vi "Event Handle Loop_Search Index.vi"(8 "error in (no error)":errorcluster, 10 "Coords":T1, 11 "QMenu Class in":refnum<class "QMenu Class.lvclass">) -> (0 "error out":errorcluster, 2 "Index":i32, 3 "QMenu Class out":refnum<class "QMenu Class.lvclass">)   [LabVIEW 2020, in "QTab.lvlib" / "QMenu Class.lvclass"]
uses:
  QMenu Class.lvclass
  <vilib>/Utility/miscctls.llb/LVPoint32TypeDef.ctl
  QMenu Class.lvclass/QMenu Class.ctl
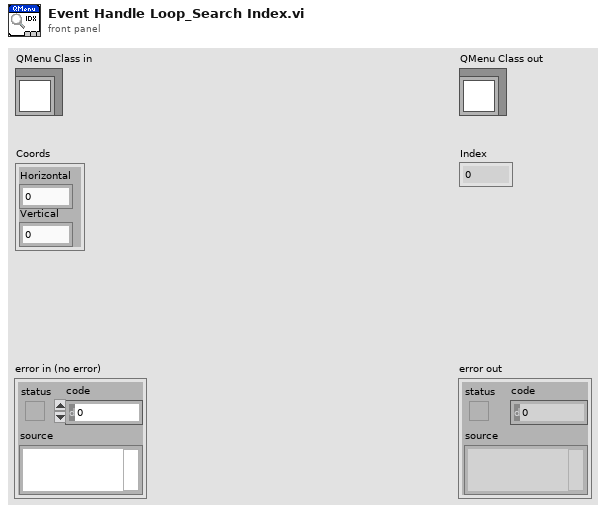
[diagram p1: front panel]
types:
  T1 = typedef "LVPoint32TypeDef.ctl" = cluster{"Horizontal":i32, "Vertical":i32}
  T2 = typedef "LVPositionTypeDef.ctl" = cluster{"Left":i32, "Top":i32}
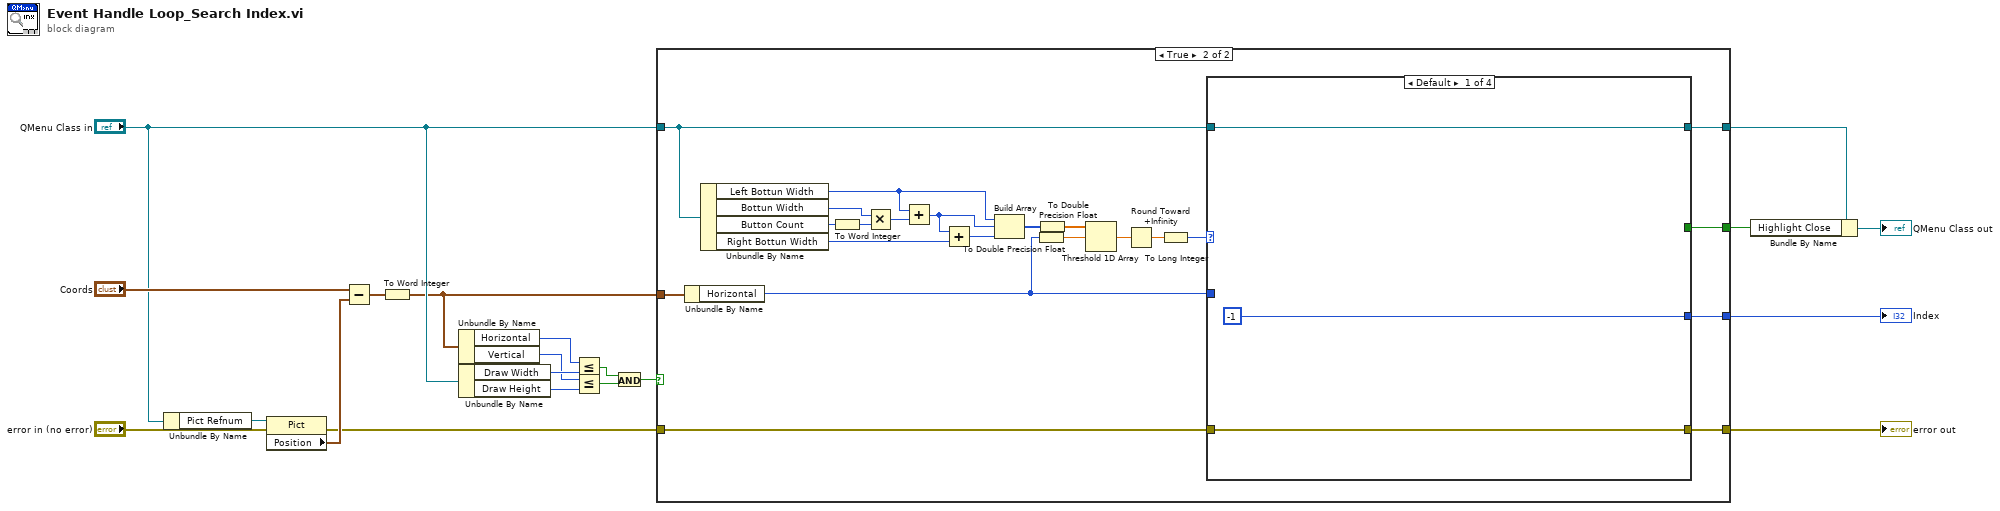
[diagram p0: block diagram]
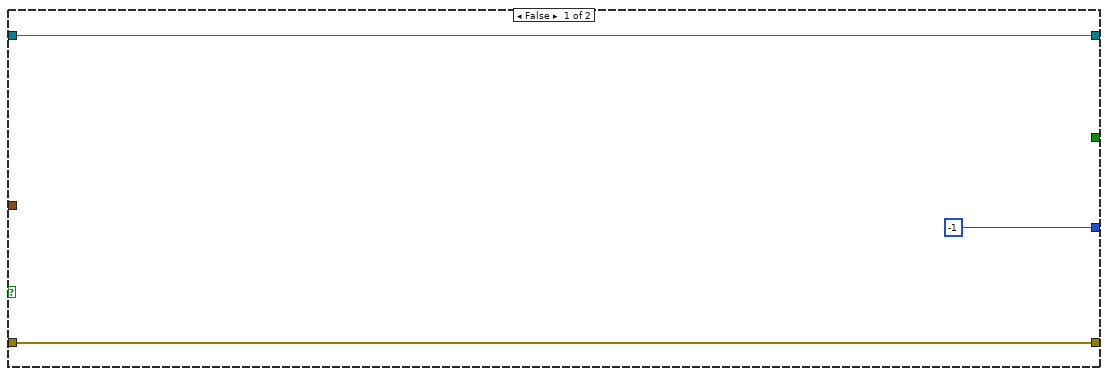
[diagram p2: hidden frame]
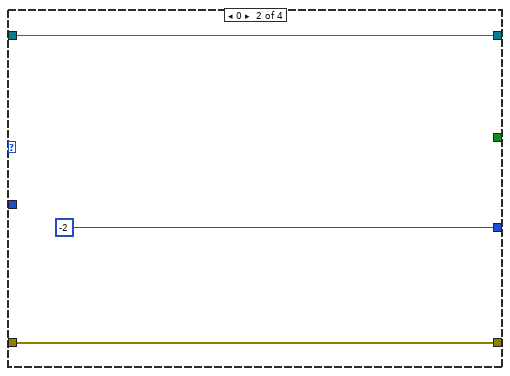
[diagram p3: hidden frame]
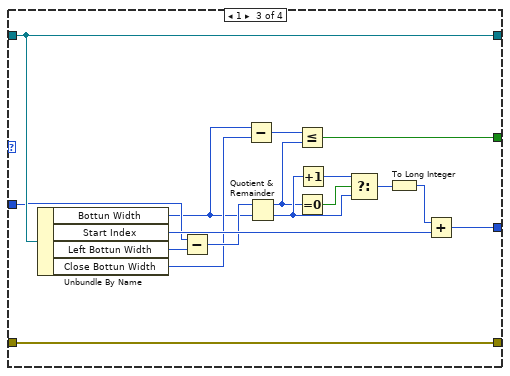
[diagram p4: hidden frame]
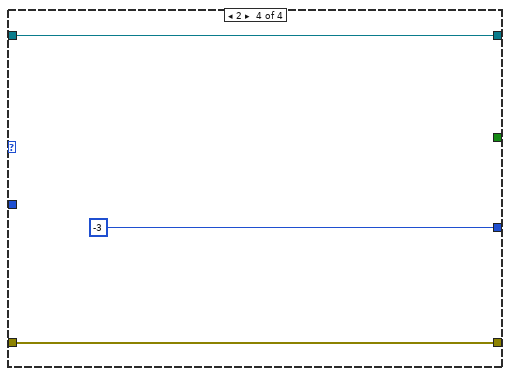
[diagram p5: hidden frame]
diagram:
  n1 = Unbundle By Name("QMenu Class in") -> ("Pict Refnum"=w20:refnum<vi>)
  n2 = property class="Pict"(reference=w20, error in="error in (no error)") -> (error out=w8:errorcluster, "Position"=w17:T2)  [unwired: 1 out]
  n3 = Subtract(x="Coords", y=w17) -> (x-y=w16:T1)
  n4 = To Word Integer(number=w16) -> (16bit integer=w5:cluster{"Horizontal":i16, "Vertical":i16})
  n5 = Unbundle By Name(w5) -> ("Horizontal"=w15:i16, "Vertical"=w12:i16)
  n6 = Unbundle By Name("QMenu Class in") -> ("Draw Width"=w14:i16, "Draw Height"=w13:i16)
  n7 = Less Or Equal?(x=w15, y=w14) -> (x <= y?=w10:bool)
  n8 = Less Or Equal?(x=w12, y=w13) -> (x <= y?=w11:bool)
  n9 = And(x=w10, y=w11) -> (x .and. y?=w7:bool)
  n10 = case shown="True" w7 {
    tunnel: "QMenu Class in" -> [w22 w28]
    tunnel: [w22 w27] -> w3
    tunnel: w8 -> [w23 w31]
    tunnel: [w23 w30] -> w6
    tunnel: w5 -> [_ w45]
    tunnel: [-1 w26] -> w4
    tunnel: [_ w24] -> w2
    frame False {
    }
    frame True {
      n11 = Unbundle By Name(w45) -> ("Horizontal"=w25:i16)
      n12 = Unbundle By Name(w28) -> ("Left Bottun Width"=w38:i16, "Bottun Width"=w44:i16, "Button Count"=w43:i32, "Right Bottun Width"=w40:i16)
      n13 = To Word Integer(number=w43) -> (16bit integer=w42:i16)
      n14 = Multiply(x=w44, y=w42) -> (x*y=w41:i16)
      n15 = Add(x=w38, y=w41) -> (x+y=w37:i16)
      n16 = Add(x=w37, y=w40) -> (x+y=w39:i16)
      n17 = Build Array(w38, w37, w39) -> (w35:i16[])
      n18 = To Double Precision Float(number=w25) -> (double precision float=w36:dbl)
      n19 = To Double Precision Float(number=w35) -> (double precision float=w34:dbl[])
      n20 = Threshold 1D Array(2:w36, 3:w34) -> (0:w33:dbl)  [unwired: 1 in]
      n21 = Round Toward +Infinity(x=w33) -> (ceil(x): smallest int >= x=w32:dbl)
      n22 = To Long Integer(number=w32) -> (32bit integer=w29:i32)
      n23 = case shown="Default" w29 {
        tunnel: w31 -> [w47 w51 w60 w69]
        tunnel: [w47 w51 w60 w69] -> w30
        tunnel: w28 -> [w48 w50 w68 w70]
        tunnel: [w48 w50 w68 w70] -> w27
        tunnel: [-1 -2 w61 -3] -> w26
        tunnel: w25 -> [_ _ w58 _]
        tunnel: [_ _ w52 _] -> w24
        frame Default {
        }
        frame 0 {
        }
        frame 1 {
          n24 = Unbundle By Name(w68) -> ("Bottun Width"=w55:i16, "Start Index"=w63:i32, "Left Bottun Width"=w59:i16, "Close Bottun Width"=w56:i16)
          n25 = Subtract(x=w58, y=w59) -> (x-y=w57:i16)
          n26 = Subtract(x=w55, y=w56) -> (x-y=w54:i16)
          n27 = Quotient & Remainder(x=w57, y=w55) -> (x-y*floor(x/y)=w53:i16, floor(x/y)=w65:i16)
          n28 = Less Or Equal?(x=w54, y=w53) -> (x <= y?=w52:bool)
          n29 = Equal To 0?(x=w53) -> (x = 0?=w67:bool)
          n30 = Increment(x=w65) -> (x+1=w66:i16)
          n31 = Select(t=w66, s=w67, f=w65) -> (s? t:f=w64:i16)
          n32 = To Long Integer(number=w64) -> (32bit integer=w62:i32)
          n33 = Add(x=w62, y=w63) -> (x+y=w61:i32)
        }
        frame 2 {
        }
      }
    }
  }
  "error out" <- w6
  "Index" <- w4
  n34 = Bundle By Name(cluster=w3, "Highlight Close"=w2) -> (→"QMenu Class out":refnum<class "QMenu Class.lvclass">)
